vi "PNA_init.vi"(2 "error in (no error)":errorcluster, 3 "PNA_control":T1={"Measurement Name (MyMeas)"="MyMeas", "Channel (1)"=1, "Start Frequency (Hz)"=1000000.0, "Stop Frequency (Hz)"=10000000000.0, "Sweep Points (201)"=201, "Measurement Parameters (S22)"="S22", "Sweep Type (0: Linear)"=0, "Sweep Generation (1: Analog)"=1, "Bandwidth (Hz)"=100000.0, "Average Count (1)"=1, "Enable Average (F: Disable)"=FALSE, "Power"={"Attenuation (0 dB)"=0.0, "Power Level (0 dBm)"=0.0, "Enable Auto Attenuation"=TRUE, "Enable RF Power"=TRUE, "Enable Power Slope"=FALSE, "Port (1)"=1, "Power Slope (0 dB/GHz)"=0.0}} {"Sweep Generation (1: Analog)" items=["Stepped", "Analog"]; "Sweep Type (0: Linear)" items=["Linear", "Logarithmic", "Power", "CW", "Segment", "Phase"]}, 4 "PNA_visa":refnum<visa-resource-name>) -> (0 "error out":errorcluster, 1 "PNA_visa_out":refnum<visa-resource-name>)   [LabVIEW 2020]
uses:
  <instrlib>/Keysight PNA Series/Keysight PNA Series.lvlib
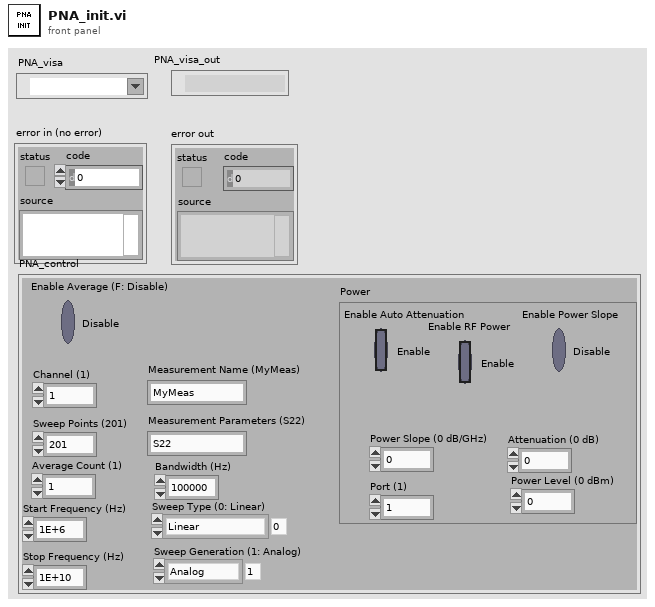
[diagram p1: front panel]
types:
  T1 = cluster{"Measurement Name (MyMeas)":string, "Channel (1)":i32, "Start Frequency (Hz)":dbl, "Stop Frequency (Hz)":dbl, "Sweep Points (201)":i32, "Measurement Parameters (S22)":string, "Sweep Type (0: Linear)":i32, "Sweep Generation (1: Analog)":i32, "Bandwidth (Hz)":dbl, "Average Count (1)":i32, "Enable Average (F: Disable)":bool, "Power":cluster{"Attenuation (0 dB)":dbl, "Power Level (0 dBm)":dbl, "Enable Auto Attenuation":bool, "Enable RF Power":bool, "Enable Power Slope":bool, "Port (1)":i32, "Power Slope (0 dB/GHz)":dbl}}
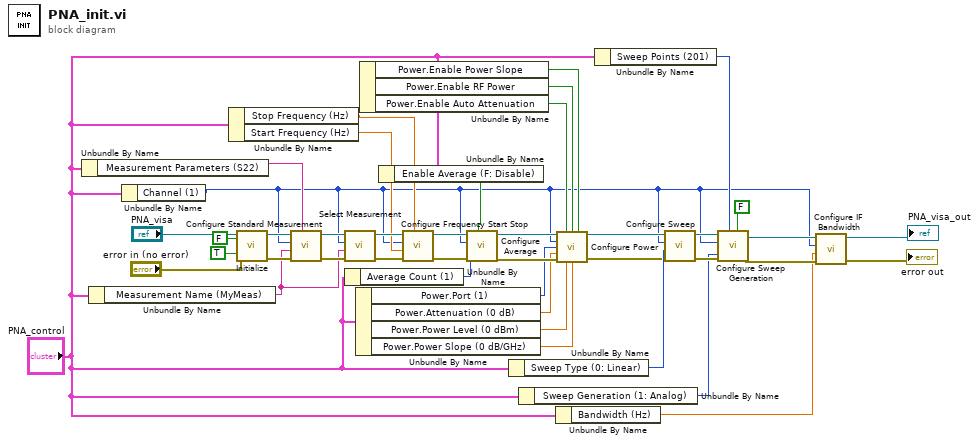
[diagram p0: block diagram]
diagram:
  n1 = Unbundle By Name("PNA_control") -> ("Measurement Parameters (S22)"=w26:string)
  n2 = Unbundle By Name("PNA_control") -> ("Measurement Name (MyMeas)"=w29:string)
  n3 = Unbundle By Name("PNA_control") -> ("Channel (1)"=w1:i32)
  n4 = Unbundle By Name("PNA_control") -> ("Stop Frequency (Hz)"=w27:dbl, "Start Frequency (Hz)"=w28:dbl)
  n5 = call <instrlib>:"Initialize.vi"("error in (no error)"="error in (no error)", "Reset (True)"=TRUE, "ID Query (True)"=FALSE, "VISA resource name"="PNA_visa") -> ("error out"=w42:errorcluster, "VISA resource name out"=w40:refnum<visa-resource-name>)  [unwired: 6 in]
  n6 = call <instrlib>:"Configure Standard Measurement.vi"("Measurement Parameters (S11)"=w26, "error in (no error)"=w42, "Measurement Name (CH1_S11_1)"=w29, "Channel (1)"=w1, "VISA resource name"=w40) -> ("error out"=w41:errorcluster, "VISA resource name out"=w39:refnum<visa-resource-name>)  [unwired: 5 in]
  n7 = call <instrlib>:"Select Measurement.vi"("error in (no error)"=w41, "Measurement Name (CH1_S11_1)"=w29, "Channel (1)"=w1, "VISA resource name"=w39) -> ("error out"=w34:errorcluster, "VISA resource name out"=w35:refnum<visa-resource-name>)  [unwired: 6 in]
  n8 = Unbundle By Name("PNA_control") -> ("Average Count (1)"=w15:i32)
  n9 = Unbundle By Name("PNA_control") -> ("Power.Port (1)"=w11:i32, "Power.Attenuation (0 dB)"=w10:dbl, "Power.Power Level (0 dBm)"=w9:dbl, "Power.Power Slope (0 dB/GHz)"=w8:dbl)
  n10 = Unbundle By Name("PNA_control") -> ("Power.Enable Power Slope"=w6:bool, "Power.Enable RF Power"=w4:bool, "Power.Enable Auto Attenuation"=w5:bool)
  n11 = Unbundle By Name("PNA_control") -> ("Enable Average (F: Disable)"=w14:bool)
  n12 = call <instrlib>:"Configure Frequency Start Stop.vi"("Stop Frequency (2E+6 Hz)"=w27, "error in (no error)"=w34, "Start Frequency (1E+6 Hz)"=w28, "Channel (1)"=w1, "VISA resource name"=w35) -> ("error out"=w16:errorcluster, "VISA resource name out"=w17:refnum<visa-resource-name>)  [unwired: 5 in]
  n13 = call <instrlib>:"Configure Average.vi"("Enable Average (F: Disable)"=w14, "error in (no error)"=w16, "Average Count (1)"=w15, "Channel (1)"=w1, "VISA resource name"=w17) -> ("error out"=w12:errorcluster, "VISA resource name out"=w13:refnum<visa-resource-name>)  [unwired: 5 in]
  n14 = Unbundle By Name("PNA_control") -> ("Sweep Type (0: Linear)"=w24:i32)
  n15 = Unbundle By Name("PNA_control") -> ("Sweep Generation (1: Analog)"=w23:i32)
  n16 = Unbundle By Name("PNA_control") -> ("Bandwidth (Hz)"=w22:dbl)
  n17 = call <instrlib>:"Configure Power.vi"("VISA resource name"=w13, "Enable Auto Attenuation (T: Enable)"=w5, "Enable RF Power (T: Enable)"=w4, "Enable Power Slope (F: Disable)"=w6, "Channel (1)"=w1, "Port (1)"=w11, "Attenuation (0 dB)"=w10, "error in (no error)"=w12, "Power Level (0 dBm)"=w9, "Power Slope (0 dB/GHz)"=w8) -> ("VISA resource name out"=w3:refnum<visa-resource-name>, "error out"=w2:errorcluster)  [unwired: 4 in]
  n18 = Unbundle By Name("PNA_control") -> ("Sweep Points (201)"=w25:i32)
  n19 = call <instrlib>:"Configure Sweep.vi"("error in (no error)"=w2, "Sweep Type (0: Linear)"=w24, "Channel (1)"=w1, "VISA resource name"=w3) -> ("error out"=w38:errorcluster, "VISA resource name out"=w37:refnum<visa-resource-name>)  [unwired: 6 in]
  n20 = call <instrlib>:"Configure Sweep Generation.vi"("Auto Sweep or Dwell Time (T: Enable)"=FALSE ("Enable Auto Sweep/Dwell Time (T: Enable)"), "Sweep Generation (1: Analog)"=w23, "Sweep Points (201)"=w25, "error in (no error)"=w38, "Channel (1)"=w1, "VISA resource name"=w37) -> ("error out"=w31:errorcluster, "VISA resource name out"=w30:refnum<visa-resource-name>)  [unwired: 4 in]
  n21 = call <instrlib>:"Configure IF Bandwidth.vi"("error in (no error)"=w31, "Bandwidth (100000 Hz)"=w22, "Channel (1)"=w1, "VISA resource name"=w30) -> ("error out"=→"error out":errorcluster, "VISA resource name out"=→"PNA_visa_out":refnum<visa-resource-name>)  [unwired: 6 in]
